vi "2131.vi"() -> ()   [LabVIEW 2014]
panel:
  in  "숫자형":dbl
  in  "불리언":bool
  in  "정지":bool
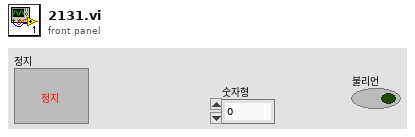
[diagram p1: front panel]
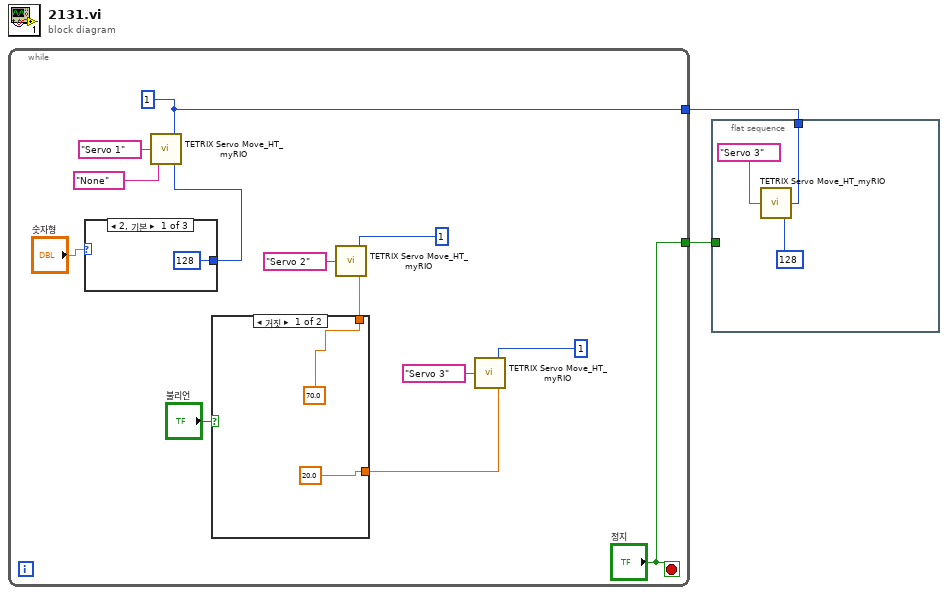
[diagram p0: block diagram]
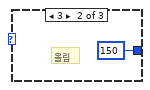
[diagram p2: hidden frame]
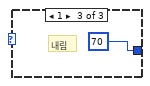
[diagram p3: hidden frame]
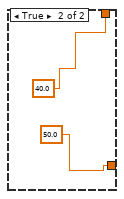
[diagram p4: hidden frame]
diagram:
  n1 = while {
    tunnel: ["정지"] -> w2
    tunnel: [w8] -> w1
    stop <- "정지" stop-if-true
    w8 = u8 1 ("Controller Daisy Chain Position (1 - 4)")
    n2 = case shown="2, 기본" "숫자형" {
      tunnel: [u8 128 ("Controller Daisy Chain Position (1 - 4)") u8 150 ("Controller Daisy Chain Position (1 - 4)") u8 70 ("Controller Daisy Chain Position (1 - 4)")] -> w3
      frame 2, Default {
      }
      frame 3 {
        # "올림"
      }
      frame 1 {
        # "내림"
      }
    }
    n3 = call <vilib>:"TETRIX Servo Move_HT_myRIO.vi"("Servo Position (0 - 255)"=w3, "Controller Daisy Chain Position (1 - 4)"=w8, "Enable Sync: Fast | Medium | Slow | None"="None", "Select Servo"="Servo 1") -> ()  [unwired: 1 in, 1 out]
    n4 = case shown="거짓" "불리언" {
      tunnel: [70.0 ("숫자형") 40.0 ("숫자형")] -> w7
      tunnel: [20.0 ("숫자형") 50.0 ("숫자형")] -> w6
      frame False {
      }
      frame True {
      }
    }
    n5 = call <vilib>:"TETRIX Servo Move_HT_myRIO.vi"("Servo Position (0 - 255)"=w7, "Controller Daisy Chain Position (1 - 4)"=u8 1, "Select Servo"="Servo 2") -> ()  [unwired: 2 in, 1 out]
    n6 = call <vilib>:"TETRIX Servo Move_HT_myRIO.vi"("Servo Position (0 - 255)"=w6, "Controller Daisy Chain Position (1 - 4)"=u8 1, "Select Servo"="Servo 3") -> ()  [unwired: 2 in, 1 out]
  }
  n7 = flat-sequence {
    tunnel: w2 -> [_]
    tunnel: w1 -> [w25]
    frame #0 {
      n8 = call <vilib>:"TETRIX Servo Move_HT_myRIO.vi"("Servo Position (0 - 255)"=u8 128, "Controller Daisy Chain Position (1 - 4)"=w25, "Select Servo"="Servo 3") -> ()  [unwired: 2 in, 1 out]
    }
  }
